vi "Create Paramaterized Executive.vi"(8 "error in (no error)":errorcluster, 10 "Create Paramaterized Executive":T1, 11 "Test Executive Builder Model in":refnum<class "Test Executive Builder Model.lvclass">) -> (0 "error out":errorcluster, 3 "Test Executive Builder Model out":refnum<class "Test Executive Builder Model.lvclass">)   [LabVIEW 2017, in "Test Executive Builder Model.lvclass"]
uses:
  Test Executive Builder Model.lvclass
  <vilib>/gpm_packages/@cs/test-executive/Source/Test Executive/TestExecutive Ref/TestExecutive Ref.lvclass
  Application Dependencies/Create Paramaterized Executive.ctl
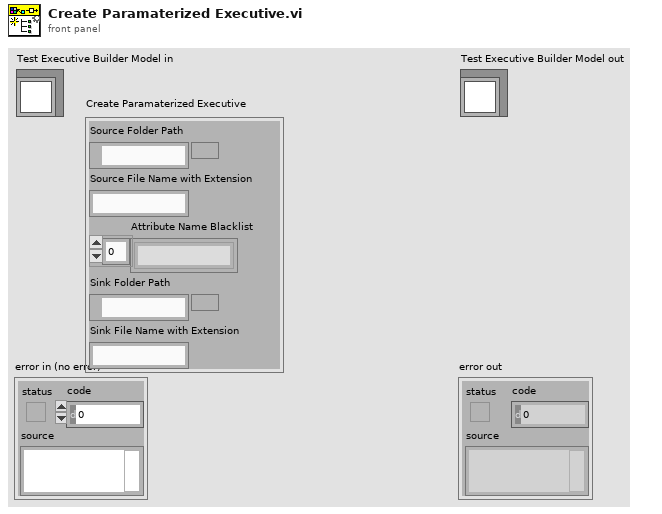
[diagram p1: front panel]
types:
  T1 = typedef "Create Paramaterized Executive.ctl" = cluster{"Source Folder Path":path, "Source File Name with Extension":string, "Attribute Name Blacklist":string[], "Sink Folder Path":path, "Sink File Name with Extension":string}
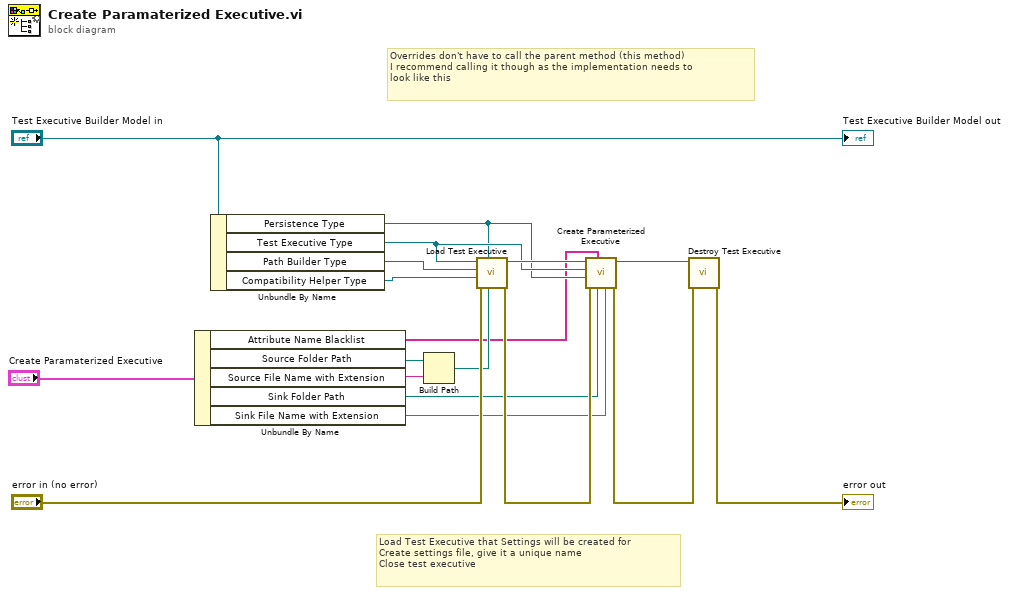
[diagram p0: block diagram]
diagram:
  # "Load Test Executive that Settings will be created for\nCreate settings file, give it a unique name\nClose test executive"
  # "Overrides don't have to call the parent method (this method)\nI recommend calling it though as the implementation needs to\nlook like this"
  n1 = Unbundle By Name("Create Paramaterized Executive") -> ("Attribute Name Blacklist"=w7:string[], "Source Folder Path"=w9:path, "Source File Name with Extension"=w8:string, "Sink Folder Path"=w2:path, "Sink File Name with Extension"=w1:string)
  n2 = Unbundle By Name("Test Executive Builder Model in") -> ("Persistence Type"=w10:refnum<class "IPersist.lvclass">, "Test Executive Type"=w11:refnum<class "ITest Executive.lvclass">, "Path Builder Type"=w17:refnum<class "IPath Builder.lvclass">, "Compatibility Helper Type"=w16:refnum<class "ICompatibility Helper.lvclass">)
  n3 = Build Path(base path=w9, name or relative path=w8) -> (appended path=w14:path)
  n4 = call <vilib>:"Load Test Executive.vi"("Folder"=w14, "Persistence in"=w10, "error in (no error)"="error in (no error)", "Compatibility Helper"=w16, "Path Builder"=w17, "Test Executive"=w11) -> ("error out"=w12:errorcluster, "Test Executive Ref out"=w13:refnum<data-value>)  [unwired: 3 in, 1 out]
  n5 = call <vilib>:"Create Parameterized Executive.vi"("File Name"=w1, "Folder"=w2, "Attribute Name Blacklist"=w7, "error in (no error)"=w12, "Persistence in"=w10, "Test Executive"=w11, "Test Executive Ref"=w13) -> ("error out"=w4:errorcluster, "Test Executive Ref out"=w5:refnum<data-value>)  [unwired: 3 in]
  n6 = call <vilib>:"Destroy Test Executive.vi"("error in (no error)"=w4, "Test Executive Ref"=w5) -> ("error out"=→"error out":errorcluster)  [unwired: 9 in]
  "Test Executive Builder Model out" <- "Test Executive Builder Model in"
